vi "lab4_sim_cp_ofdm_transceiver.vi"() -> ()   [LabVIEW 2014]
uses:
  <vilib>/addons/Modulation/Digital/General/MT Generate Bits (Galois, PN Order).vi
  <vilib>/Analysis/2dsp.llb/Inverse Complex FFT.vi
  <vilib>/Analysis/2dsp.llb/Complex FFT.vi
  <vilib>/Analysis/5stat.llb/RMS (DBL).vi
  <vilib>/addons/Modulation/Digital/Support/Common/Validators/mod_Generate Bits Validate.vi
  <vilib>/addons/Modulation/Analog/support/mod_Set Error Source.vi
  <vilib>/addons/Modulation/Digital/General/MT Generate QAM System Parameters(M).vi
  <vilib>/addons/Modulation/Digital/General/subVIs/mod_Generate Bits PN Sequence.vi
  <vilib>/addons/Modulation/Digital/General/MT Map Bits to QAM Symbols.vi
  <vilib>/gmath/statdist.llb/Normal Random.vi
  <vilib>/addons/Modulation/Digital/General/MT Map QAM Symbols to Bits.vi
  <vilib>/Analysis/NI_AALPro.lvlib
  <vilib>/addons/Modulation/niDMT.lvlib
  <vilib>/gmath/NI_Gmath.lvlib
panel:
  out "Phase":dbl[](graph)
  out "Amplitude":dbl[](graph)
  out "Average PAPR":dbl
  out "PAPR":dbl
  out "Error bits":i32
  out "Bit compare":bool[](array[boolean])
  out "BER":dbl
  in  "millisecond multiple":u32=20
  out "output bit stream 2":i8[](array[numeric]) caption="Transmit output bit stream"
  out "output bit stream":i8[](array[numeric]) caption="Received output bit stream"
  in  "M-QAM (16)":i32=16
  out "Transmit FFT (Magnitude)":dbl[](graph)
  out "Receiver FFT (Magnitude)":dbl[](graph)
  out "RX constellation":cdb[](graph)
  in  "pilot carrier":i32=32
  in  "message carrier":i32=120
  out "eb/n0 (dB)":dbl=38.96307662438871
  in  "Symbol energy es/n0(db)":dbl=50.0 format="%#_13g"
  in  "stop":bool
  in  "cyclic prefix":i32=64
  in  "FFT size":i32=256
  in  "ofdm symbols":i32=10
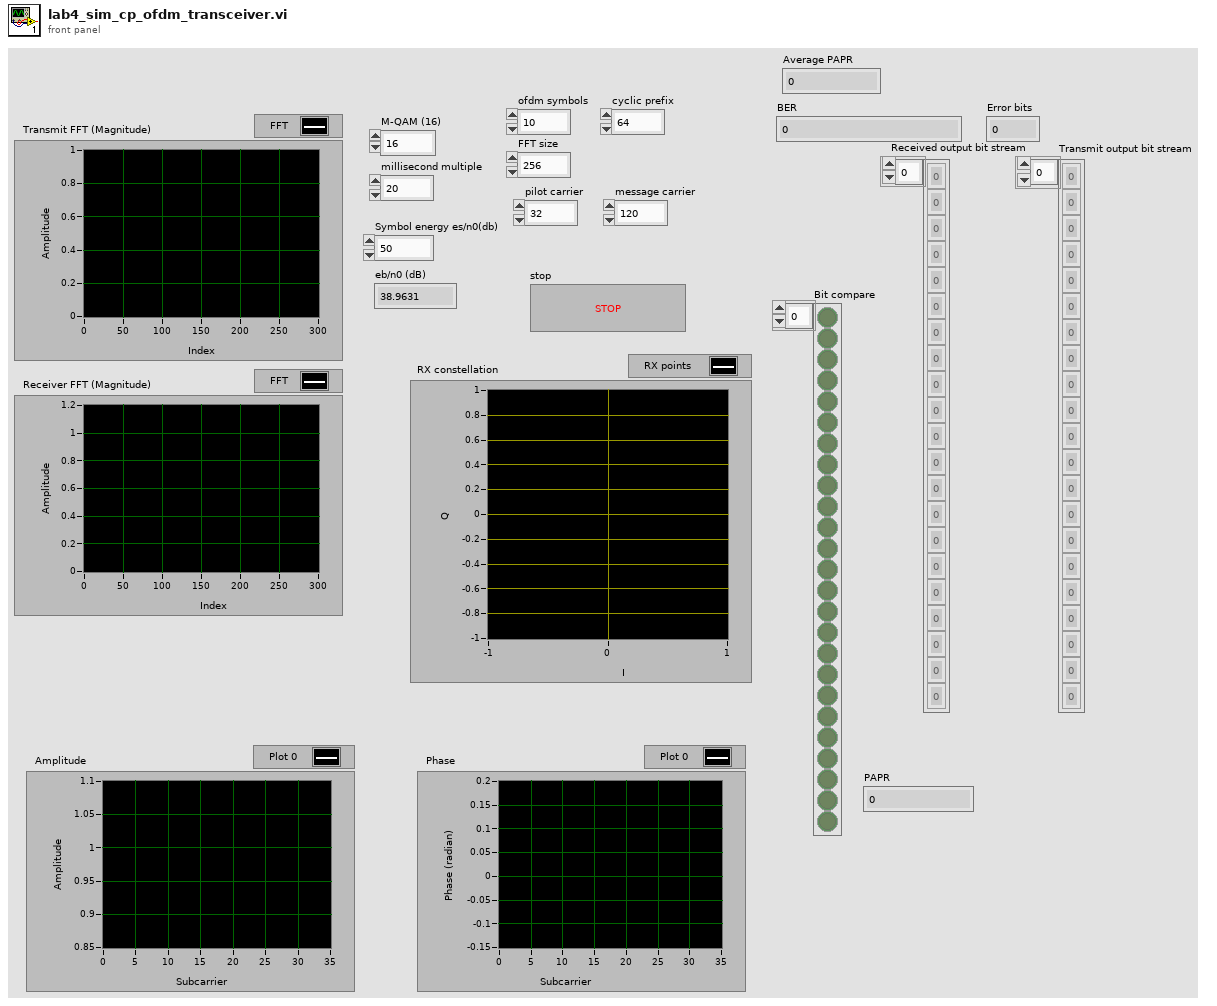
[diagram p1: front panel]
types:
  T1 = cluster{"samples per symbol (16)":i32, "symbol map":cdb[]}
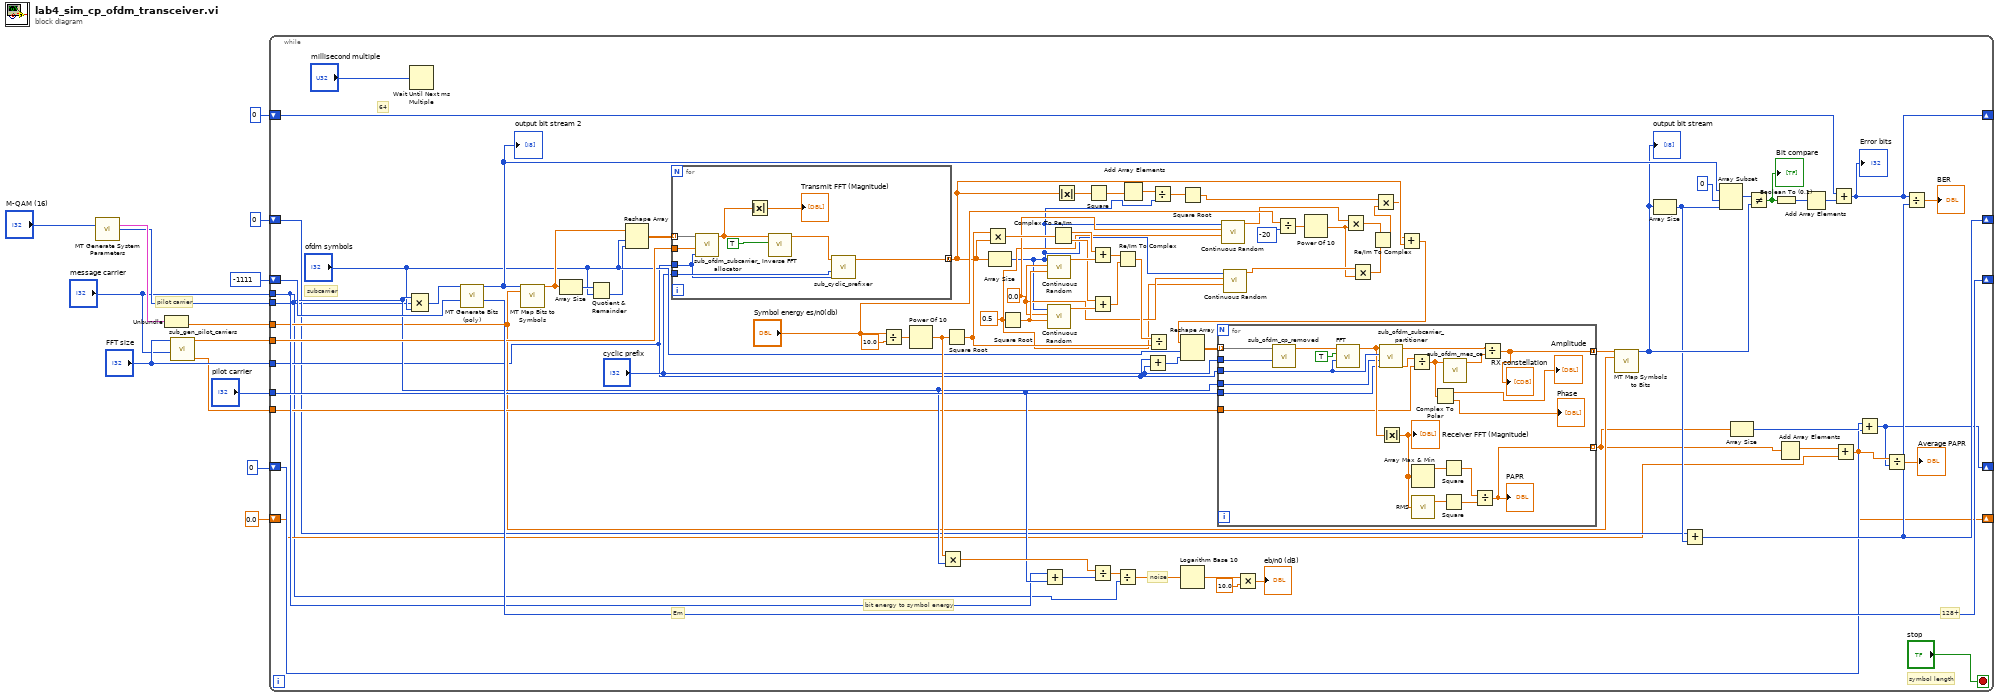
[diagram p0: block diagram]
diagram:
  # "pilot carrier"
  n1 = call-poly <vilib>:"MT Generate System Parameters.vi"("M-QAM (16)"="M-QAM (16)") -> ("QAM system parameters"=w11:T1, "bits per symbol"=w9:i32)  [unwired: 12 in, 1 out]
  n2 = Unbundle(w11) -> ("symbol map"=w10:cdb[])  [unwired: 1 out]
  n3 = call "sub_gen_pilot_carriers.vi"("message carrier"="message carrier", "FFT size"="FFT size") -> ("RX pilot carriers"=w4:cdb[], "TX pilot carriers"=w3:cdb[])  [unwired: 8 in]
  n4 = while {
    tunnel: w9 -> [w35]
    shift-right: [w95] -> _
    shift-left: -1111 ("seed out") -> [w96]
    tunnel: w3 -> [w80]
    tunnel: "pilot carrier" -> [w78]
    tunnel: "message carrier" -> [w77]
    tunnel: "FFT size" -> [w61]
    tunnel: w4 -> [w76]
    tunnel: w10 -> [w75]
    shift-right: [w46] -> _
    shift-left: 0 -> [w49]
    shift-right: [w45] -> _
    shift-left: 0 -> [w47]
    shift-right: [w37] -> _
    shift-left: 0 -> [w41]
    shift-right: [w38] -> _
    shift-left: 0.0 -> [w39]
    stop <- "stop" stop-if-true
    w33 = 0.5 ("std")
    w34 = 0.0 ("mean")
    # "symbol length"
    # "bit energy to symbol energy"
    # "noise"
    # "128+"
    # "subcarrier"
    # "Em"
    # "64"
    n5 = Wait Until Next ms Multiple(millisecond multiple="millisecond multiple") -> ()  [unwired: 1 out]
    n6 = Compound Arithmetic op=MULTIPLY(w77, w35, "ofdm symbols") -> (w72:i32)
    n7 = call-poly <vilib>:"MT Generate Bits (poly).vi"("total bits (128)"=w72, "seed in (0xD6BF7DF2)"=w96) -> ("output bit stream"=w70:i8[], "seed out"=w95:i32)  [unwired: 11 in, 1 out]
    "output bit stream 2" <- w70
    n8 = call-poly <vilib>:"MT Map Bits to Symbols.vi"("input bit stream"=w70, "symbol map"=w75) -> ("symbols"=w82:cdb[])  [unwired: 12 in, 1 out]
    n9 = Array Size(array=w82) -> (size(s)=w94:i32)
    n10 = Quotient & Remainder(x=w94, y="ofdm symbols") -> (floor(x/y)=w64:i32)  [unwired: 1 out]
    n11 = Reshape Array(w82, "ofdm symbols", w64) -> (w81:cdb[][])
    n12 = for {
      tunnel: w81 -> [w127] mode=indexing
      tunnel: w80 -> [w126]
      tunnel: w61 -> [w122]
      tunnel: "cyclic prefix" -> [w123]
      tunnel: [w121] -> w24 mode=concatenating
      n13 = call "sub_ofdm_subcarrier_allocator.vi"("fft size"=w122, "pilot symbol"=w126, "message symbol"=w127) -> ("OFDM symbol"=w120:cdb[])  [unwired: 8 in]
      n14 = Absolute Value(x=w120) -> (abs(x)=→"Transmit FFT (Magnitude)":dbl[])
      n15 = call-poly <vilib>:"Inverse FFT.vi"("shift?"=TRUE, "FFT {X}"=w120) -> ("X"=w124:cdb[])  [unwired: 8 in, 1 out]
      n16 = call "sub_cyclic_prefixer.vi"("FFT size"=w122, "CP length"=w123, "time_samples"=w124) -> ("cp ofdm symbol"=w121:cdb[])  [unwired: 8 in]
    }
    n17 = Divide(x="Symbol energy es/n0(db)", y=10.0) -> (x/y=w90:dbl)
    n18 = Power Of 10(x=w90) -> (10^x=w86:dbl)
    n19 = Multiply(x=w86, y=w77) -> (x*y=w85:dbl)
    n20 = Square Root(x=w86) -> (sqrt(x)=w51:dbl)
    n21 = Multiply(x=w51, y=w24) -> (x*y=w59:cdb[])
    n22 = Array Size(array=w24) -> (size(s)=w19:i32)
    n23 = Square Root(x=w33) -> (sqrt(x)=w44:dbl)
    n24 = Add(x=w77, y=w78) -> (x+y=w79:i32)
    n25 = call-poly <vilib>:"Continuous Random.vi"("std"=w44, "mean"=w34, "samples"=w19) -> ("normal random data"=w57:dbl[])  [unwired: 7 in, 1 out]
    n26 = call-poly <vilib>:"Continuous Random.vi"("std"=w44, "mean"=w34, "samples"=w19) -> ("normal random data"=w55:dbl[])  [unwired: 7 in, 1 out]
    n27 = Complex To Re/Im(x + iy=w59) -> (x=w58:dbl[], y=w56:dbl[])
    n28 = Absolute Value(x=w24) -> (abs(x)=w22:dbl[])
    n29 = Square(x=w22) -> (x^2=w21:dbl[])
    n30 = Add(x=w58, y=w57) -> (x+y=w54:dbl[])
    n31 = Add(x=w56, y=w55) -> (x+y=w53:dbl[])
    n32 = Divide(x=w85, y=w79) -> (x/y=w84:dbl)
    n33 = Re/Im To Complex(1:w53, 2:w54) -> (0:w52:cdb[])
    n34 = Divide(x=w84, y=w35) -> (x/y=w83:dbl)
    n35 = Add Array Elements(numeric array=w21) -> (sum=w20:dbl)
    n36 = Add(x=w61, y="cyclic prefix") -> (x+y=w60:i32)
    n37 = Divide(x=w52, y=w51) -> ()  [unwired: 1 out]
    n38 = Divide(x=w20, y=w19) -> (x/y=w18:dbl)
    n39 = Square Root(x=w18) -> (sqrt(x)=w17:dbl)
    n40 = Logarithm Base 10(1:w83) -> (0:w89:dbl)
    n41 = call-poly <vilib>:"Continuous Random.vi"("std"=w33, "mean"=w34, "samples"=w19) -> ("normal random data"=w28:dbl[])  [unwired: 7 in, 1 out]
    n42 = call-poly <vilib>:"Continuous Random.vi"("std"=w33, "mean"=w34, "samples"=w19) -> ("normal random data"=w29:dbl[])  [unwired: 7 in, 1 out]
    n43 = Multiply(x=w89, y=10.0) -> (x*y=→"eb/n0 (dB)":dbl)
    n44 = Divide(x="Symbol energy es/n0(db)", y=-20) -> (x/y=w30:dbl)
    n45 = Power Of 10(x=w30) -> (10^x=w27:dbl)
    n46 = Multiply(x=w28, y=w27) -> (x*y=w26:dbl[])
    n47 = Multiply(x=w29, y=w27) -> (x*y=w25:dbl[])
    n48 = Re/Im To Complex(1:w25, 2:w26) -> (0:w16:cdb[])
    n49 = Multiply(x=w17, y=w16) -> (x*y=w15:cdb[])
    n50 = Add(x=w15, y=w24) -> (x+y=w23:cdb[])
    n51 = Reshape Array(w23, "ofdm symbols", w60) -> (w63:cdb[][])
    n52 = for {
      tunnel: w63 -> [w118] mode=indexing
      tunnel: "cyclic prefix" -> [w117]
      tunnel: w61 -> [w114]
      tunnel: [w97] -> w66 mode=concatenating
      tunnel: w77 -> [w112]
      tunnel: w78 -> [w111]
      tunnel: w76 -> [w101]
      tunnel: [w105] -> w43 mode=indexing
      n53 = call "sub_ofdm_cp_removed.vi"("CP length"=w117, "time ofdm symbol"=w118) -> ("cp removed ofdm symbol"=w115:cdb[])  [unwired: 9 in]
      n54 = call-poly <vilib>:"FFT.vi"("FFT size"=w114, "shift?"=TRUE, "X"=w115) -> ("FFT {X}"=w113:cdb[])  [unwired: 7 in, 1 out]
      n55 = call "sub_ofdm_subcarrier_partitioner.vi"("pilot carrier"=w111, "message carrier"=w112, "FFT size"=w114, "received symbol"=w113) -> ("pilot subcarriers"=w100:cdb[], "message subcarriers"=w99:cdb[])  [unwired: 6 in]
      n56 = Absolute Value(x=w113) -> (abs(x)=w110:dbl[])
      "Receiver FFT (Magnitude)" <- w110
      n57 = Divide(x=w100, y=w101) -> (x/y=w104:cdb[])
      n58 = Array Max & Min(array=w110) -> (max value=w109:dbl)  [unwired: 3 out]
      n59 = call-poly <vilib>:"RMS.vi"("X"=w110) -> ("rms value"=w108:dbl)  [unwired: 1 out]
      n60 = Complex To Polar(r * e^(i*theta)=w104) -> (r=→"Amplitude":dbl[], theta=→"Phase":dbl[])
      n61 = Square(x=w109) -> (x^2=w107:dbl)
      n62 = Square(x=w108) -> (x^2=w106:dbl)
      n63 = call "sub_ofdm_mes_ce.vi"("ZF channel estimates"=w104) -> ("interpolated mes carrier CE"=w98:cdb[])  [unwired: 10 in]
      n64 = Divide(x=w107, y=w106) -> (x/y=w105:dbl)
      "PAPR" <- w105
      n65 = Divide(x=w99, y=w98) -> (x/y=w97:cdb[])
      "RX constellation" <- w97
    }
    n66 = call-poly <vilib>:"MT Map Symbols to Bits.vi"("symbols"=w66, "symbol map"=w75) -> ("output bit stream"=w69:i8[])  [unwired: 12 in, 1 out]
    "output bit stream" <- w69
    n67 = Array Size(array=w69) -> (size(s)=w48:i32)
    n68 = Add(x=w47, y=w48) -> (x+y=w45:i32)
    n69 = Array Subset(array=w70, index=0, length=w48) -> (w67:i8[])
    n70 = Array Size(array=w43) -> (size(s)=w42:i32)
    n71 = Not Equal?(x=w67, y=w69) -> (x != y?=w74:bool[])
    "Bit compare" <- w74
    n72 = Boolean To (0,1)(Boolean=w74) -> (0, 1=w73:i16[])
    n73 = Add Array Elements(numeric array=w43) -> (sum=w40:dbl)
    n74 = Add Array Elements(numeric array=w73) -> (sum=w50:i16)
    n75 = Add(x=w49, y=w50) -> (x+y=w46:i32)
    "Error bits" <- w46
    n76 = Add(x=w40, y=w39) -> (x+y=w38:dbl)
    n77 = Add(x=w42, y=w41) -> (x+y=w37:i32)
    n78 = Divide(x=w38, y=w37) -> (x/y=→"Average PAPR":dbl)
    n79 = Divide(x=w46, y=w45) -> (x/y=→"BER":dbl)
  }
